vi "DTACQ - Querry Status.vi"(8 "error in":errorcluster, 11 "Address":string) -> (0 "error out":errorcluster, 1 "Analog Out Busy":bool, 2 "Module Carrier Status":T1, 5 "Timed Out":bool=TRUE)   [LabVIEW 2017, in "Communications Library.lvlib"]
doc: "Querries the status of the DTACQ device.\n\nThe status of both the module carrier and the analog out module are querried."
uses:
  Communications Library.lvlib
  Typedefs/DTACQ Module Carrier Status.ctl
  Typedefs/DTACQ Status--Enum.ctl
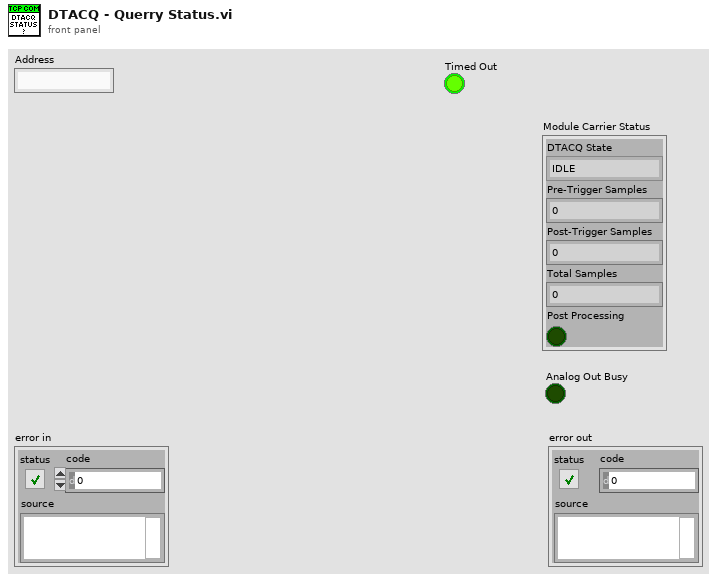
[diagram p1: front panel]
types:
  T1 = typedef "Communications Library.lvlib/DTACQ Module Carrier Status.ctl" = cluster{"DTACQ State":T2, "Pre-Trigger Samples":i32, "Post-Trigger Samples":i32, "Total Samples":i32, "Post Processing":bool}
  T2 = typedef "Communications Library.lvlib/DTACQ Status--Enum.ctl" = enum16{"IDLE", "ARM", "RUN_PRE-TRIGGER", "RUN_POST-TRIGGER", "POST_PROCESS", "CLEANUP"}
  T3 = typedef "Communications Library.lvlib/DTACQ Connection Data--Cluster.ctl" = cluster{"Description":string, "Address":string, "Port":u16, "timeout (ms)":i32, "Termination Character":string, "TCP Connection Reference":refnum<k5>, "Open Connection":bool}
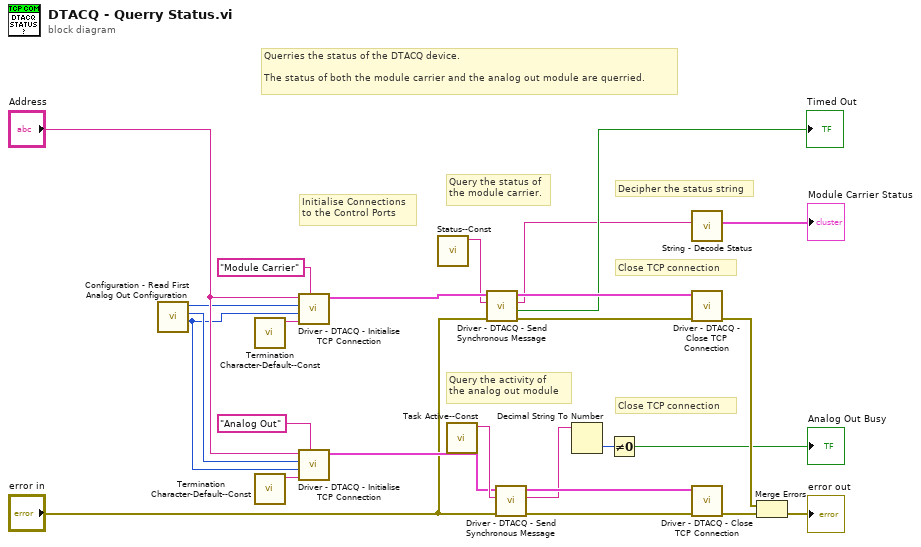
[diagram p0: block diagram]
diagram:
  # "Querries the status of the DTACQ device.\n\nThe status of both the module carrier and the analog out module are querried."
  # "Close TCP connection"
  # "Close TCP connection"
  # "Decipher the status string"
  # "Query the activity of\nthe analog out module"
  # "Query the status of\nthe module carrier."
  # "Initialise Connections\nto the Control Ports"
  n1 = call "Configuration - Read First Analog Out Configuration.vi"() -> ("Timeout (ms)"=w1:i32, "Analog Out Control Port"=w2:i32, "Carrier Control Port"=w3:i32)  [unwired: 7 in, 2 out]
  n2 = call "Termination Character-Default--Const.vi"() -> ("Termination Character"=w21:string)  [unwired: 11 in]
  n3 = call "Termination Character-Default--Const.vi"() -> ("Termination Character"=w19:string)  [unwired: 11 in]
  n4 = call "Driver - DTACQ - Initialise TCP Connection.vi"("Description"="Module Carrier", "Termination Character"=w21, "timeout (ms)"=w1, "Port"=w3, "Address"="Address") -> ("DTACQ Connection Data Out"=w15:T3)  [unwired: 6 in]
  n5 = call "Driver - DTACQ - Initialise TCP Connection.vi"("Description"="Analog Out", "Termination Character"=w19, "timeout (ms)"=w1, "Port"=w2, "Address"="Address") -> ("DTACQ Connection Data Out"=w13:T3)  [unwired: 6 in]
  n6 = call "Status--Const.vi"() -> ("Status Command"=w14:string)  [unwired: 11 in]
  n7 = call "Task Active--Const.vi"() -> ("Task Active Command"=w18:string)  [unwired: 11 in]
  n8 = call "Driver - DTACQ - Send Synchronous Message.vi"("error in"="error in", "Message to Send"=w14, "DTACQ Connection Data In"=w15) -> ("error out"=w12:errorcluster, "Timed Out"=→"Timed Out":bool, "Read String"=w4:string, "DTACQ Connection Data Out"=w7:T3)  [unwired: 5 in]
  n9 = call "Driver - DTACQ - Send Synchronous Message.vi"("error in"="error in", "Message to Send"=w18, "DTACQ Connection Data In"=w13) -> ("error out"=w24:errorcluster, "Read String"=w10:string, "DTACQ Connection Data Out"=w25:T3)  [unwired: 5 in, 1 out]
  n10 = Decimal String To Number(string=w10) -> (number=w9:i32)  [unwired: 2 in, 1 out]
  n11 = Not Equal To 0?(x=w9) -> (x != 0?=→"Analog Out Busy":bool)
  n12 = call "String - Decode Status.vi"("Status Response String"=w4) -> ("Module Carrier Status"=→"Module Carrier Status":T1)  [unwired: 9 in, 1 out]
  n13 = call "Driver - DTACQ - Close TCP Connection.vi"("error in"=w12, "DTACQ Connection Data In"=w7) -> ("error out"=w16:errorcluster)  [unwired: 8 in, 1 out]
  n14 = call "Driver - DTACQ - Close TCP Connection.vi"("error in"=w24, "DTACQ Connection Data In"=w25) -> ("error out"=w17:errorcluster)  [unwired: 8 in, 1 out]
  n15 = Merge Errors(w16, w17) -> (→"error out":errorcluster)
